vi "Flatten to YAML.vi"(8 "error in (no error)":errorcluster, 11 "Anything":variant) -> (0 "error out":errorcluster, 3 "YAML String":string)   [LabVIEW 2015, in "YAML Parser.lvlib"]
uses:
  YAML Parser.lvlib
  <vilib>/Utility/Data Type/NI_Data Type.lvlib
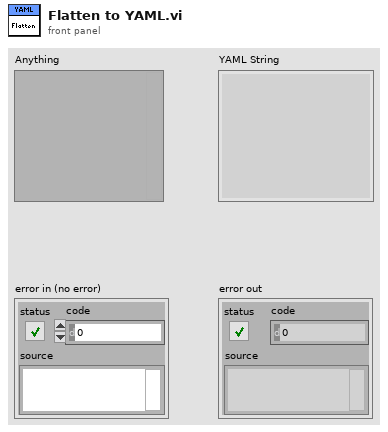
[diagram p1: front panel]
types:
  T1 = typedef "NI_Data Type.lvlib/Data Type.ctl" = enum8{"Invalid Type", "Void", "I8", "I16", "I32", "I64", "U8", "U16", "U32", "U64", "Single Float", "Double Float", "Extended Float", "Single Complex", "Double Complex", "Extended Complex", "Enum U8", "Enum U16", "Enum U32", "Enum U64", "Single Float With Unit", "Double Float With Unit", "Extended Float With Unit", "Single Complex with Unit", "Double Complex with Unit", "Extended Complex with Unit", "Boolean", "String", "Path", "Picture", "Tag", "Array", "Cluster", "Variant", "LV Variant", "Waveform", "Timestamp", "Digital Waveform", "Digital Data", "ExpressData", "Refnum", "External Data", "VI", "Poly VI", "LabVIEW Class Instance", "Fixed Point"}
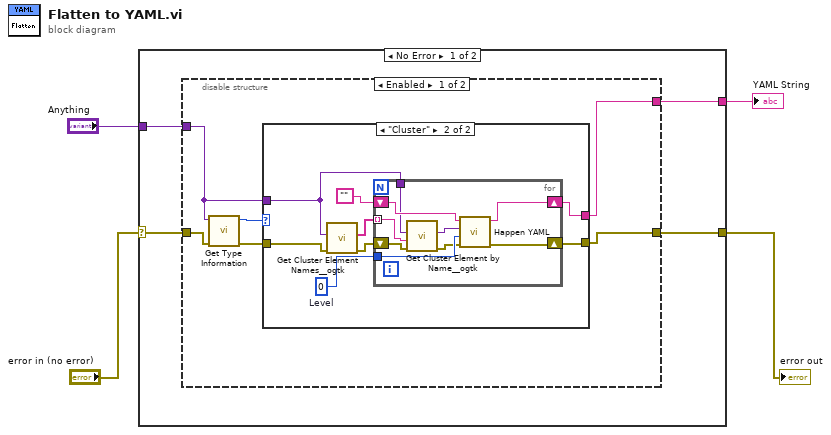
[diagram p0: block diagram]
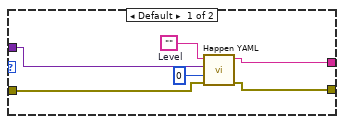
[diagram p2: hidden frame]
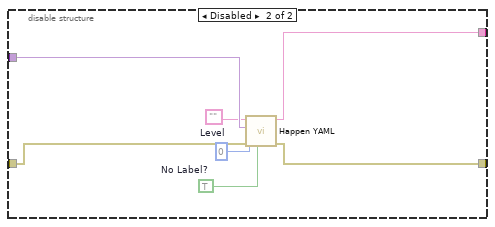
[diagram p3: hidden frame]
diagram:
  n1 = case shown="No Error" "error in (no error)" {
    selector: "error in (no error)" -> [w8 w45]
    tunnel: [w7 w45] -> w3
    tunnel: "Anything" -> [w6 _]
    tunnel: [w5 _] -> w1
    frame No Error {
      n2 = disable-structure shown="Enabled" {
        disable-tunnel: w8 -> [w12 w44]
        disable-tunnel: [w11 w43] -> w7
        disable-tunnel: w6 -> [w10 w42]
        disable-tunnel: [w9 w38] -> w5
        frame Enabled {
          n3 = call <vilib>:"Get Type Information.vi"("error in (no error)"=w12, "Variant"=w10) -> ("error out"=w13:errorcluster, "Type"=w14:T1)  [unwired: 5 in, 3 out]
          n4 = case shown="\"Cluster\"" w14 {
            tunnel: w13 -> [w18 w24]
            tunnel: w10 -> [w16 w21]
            tunnel: [w17 w28] -> w11
            tunnel: [w15 w27] -> w9
            frame Default {
              w19 = u32 0  # Level
              n5 = call "Happen YAML.vi"("error in (no error)"=w18, "Level"=w19, "Anything"=w16, "YAML String in"="") -> ("error out"=w17:errorcluster, "YAML String out"=w15:string)  [unwired: 6 in]
            }
            frame "Cluster" {
              w25 = u32 0  # Level
              n6 = call <userlib>:"Get Cluster Element Names__ogtk.vi"("error in (no error)"=w24, "Cluster"=w21) -> ("error out"=w23:errorcluster, "Element Names"=w22:string[])  [unwired: 8 in]
              n7 = for {
                tunnel: w22 -> [w30] mode=indexing
                shift-right: [w37] -> w28
                shift-left: w23 -> [w33]
                shift-right: [w34] -> w27
                shift-left: "" -> [w35]
                tunnel: w25 -> [w36]
                tunnel: w21 -> [w31]
                n8 = call <userlib>:"Get Cluster Element by Name__ogtk.vi"("error in (no error)"=w33, "Element Name"=w30, "Cluster"=w31) -> ("error out"=w32:errorcluster, "VElement"=w29:variant)  [unwired: 6 in, 1 out]
                n9 = call "Happen YAML.vi"("error in (no error)"=w32, "Level"=w36, "Anything"=w29, "YAML String in"=w35) -> ("error out"=w37:errorcluster, "YAML String out"=w34:string)  [unwired: 6 in]
              }
            }
          }
        }
        frame Disabled {
          w39 = TRUE  # No Label?
          w40 = u32 0  # Level
          n10 = call "Happen YAML.vi"("No Label?"=w39, "error in (no error)"=w44, "Level"=w40, "Anything"=w42, "YAML String in"="") -> ("error out"=w43:errorcluster, "YAML String out"=w38:string)  [unwired: 5 in]
        }
      }
    }
    frame Error {
    }
  }
  "error out" <- w3
  "YAML String" <- w1
